vi "UpdateCVTFromSettingsCluster.vi"(8 "error in":errorcluster, 10 "SelectedProperty.Hierarchy":string[](array[string]), 11 "SettingsCluster":variant) -> (0 "error out":errorcluster)   [LabVIEW 2020]
uses:
  OnOffTypeDef.ctl
  UtilsLib/ClusterManipulation/GetClusterElementByName(Variant).vi
  UtilsLib/ClusterManipulation/GetClusterElementByName(DBL).vi
  CompressAndUpdate(Poly)/CompressAndUpdate(Enum).vi
  CompressAndUpdate(Poly)/CompressAndUpdate(Numeric).vi
  CompressAndUpdate(Poly)/CompressAndUpdate(String).vi
  CompressAndUpdate(Poly)/CompressAndUpdate(Path).vi
  UtilsLib/ClusterManipulation/GetClusterElementByName.lvlib
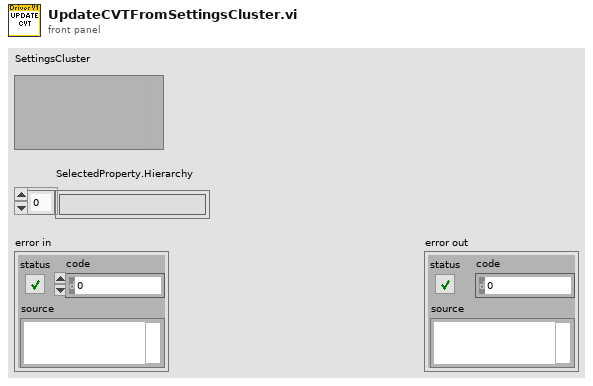
[diagram p1: front panel]
types:
  T1 = typedef "OnOffTypeDef.ctl" = enum16{"off", "on"}
  T2 = typedef "Type Descriptor Enumeration__ogtk.ctl" = enum8{"<Null>", "I8", "I16", "I32", "I64", "U8", "U16", "U32", "U64", "SGL", "DBL", "EXT", "CSG", "CDB", "CXT", "0x0F", "0x10", "0x11", "0x12", "0x13", "0x14", "Enum U8", "Enum U16", "Enum U32", "Enum U64", "SGL PQ", "DBL PQ", "EXT PQ", "CSG PQ", "CDB PQ", "CXT PQ", "0x1F", "0x20", "Boolean", "0x22", "0x23", "0x24", "0x25", "0x26", "0x27", "0x28", "0x29", "0x2A", "0x2B", "0x2C", "0x2D", "0x2E", "0x2F", "String", "0x31", "Path", "Pict", "0x34", "0x35", "0x36", "DAQ", "0x38", "0x39", "0x3A", "0x3B", "0x3C", "0x3D", "0x3E", "0x3F", "Array", "0x41", "0x42", "0x43", "0x44", "0x45", "0x46", "0x47", "0x48", "0x49", "0x4A", "0x4B", "0x4C", "0x4D", "0x4E", "0x4F", "Cluster", "0x51", "0x52", "Variant", "Waveform", "0x55", "0x56", "0x57", "0x58", "0x59", "0x5A", "0x5B", "0x5C", "0x5D", "0x5E", "0x5F", "0x60", "0x61", "0x62", "0x63", "0x64", "0x65", "0x66", "0x67", "0x68", "0x69", "0x6A", "0x6B", "0x6C", "0x6D", "0x6E", "0x6F", "Refnum"}
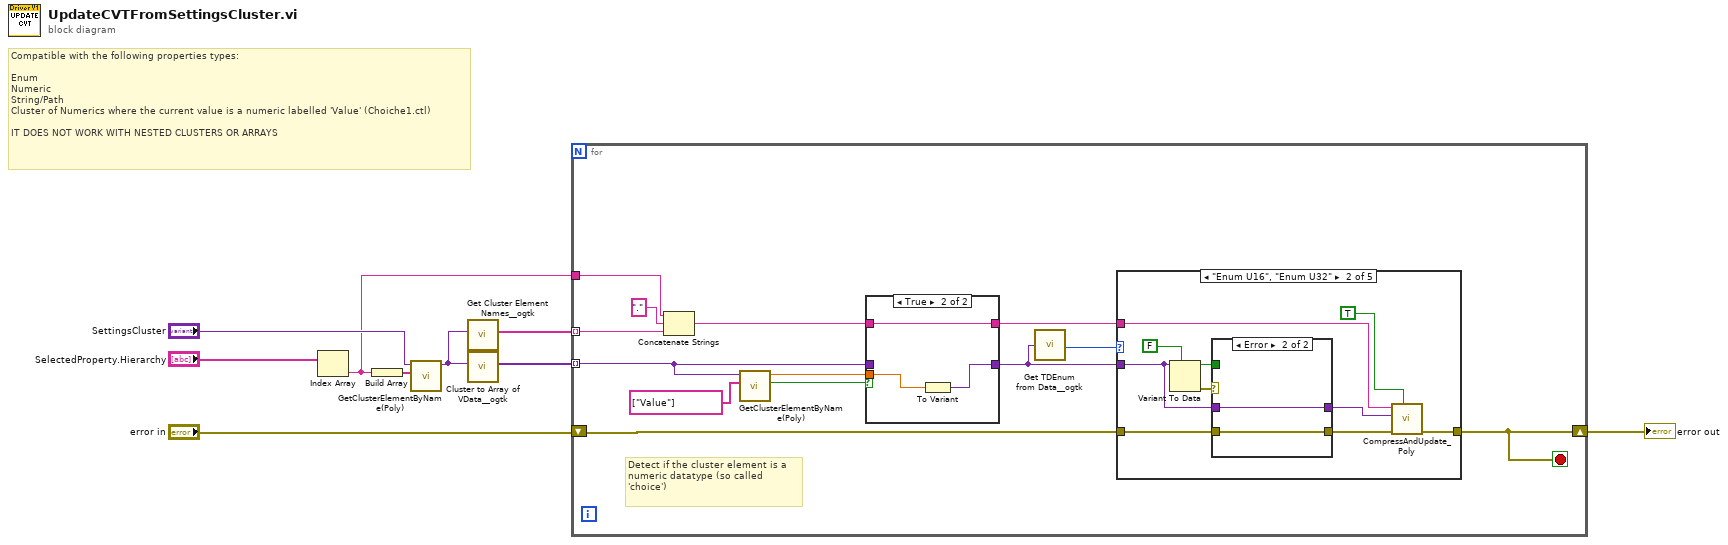
[diagram p0: block diagram]
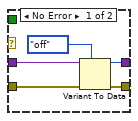
[diagram p3: hidden frame]
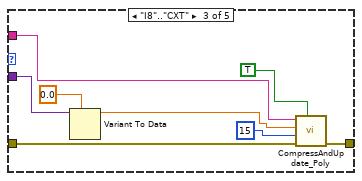
[diagram p4: hidden frame]
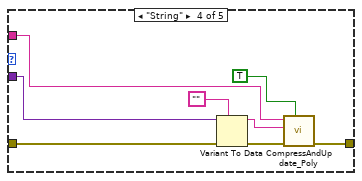
[diagram p5: hidden frame]
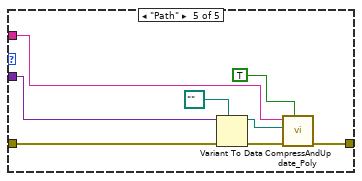
[diagram p6: hidden frame]
diagram:
  # "Compatible with the following properties types:\n\nEnum\nNumeric\nString/Path\nCluster of Numerics where the current value is a numeric labelled 'Value' (Choiche1.ctl)\n\nIT DOES NOT WORK WITH NESTED CLUSTERS OR ARRAYS"
  n1 = Index Array(array="SelectedProperty.Hierarchy") -> (element=w1:string)  [unwired: 1 in]
  n2 = Build Array(w1) -> (w2:string[])
  n3 = call-poly "GetClusterElementByName(Poly).vi"("ElementHierarchy"=w2, "Cluster"="SettingsCluster") -> ("Element"=w7:variant)  [unwired: 8 in, 1 out]
  n4 = call <userlib>:"Get Cluster Element Names__ogtk.vi"("Cluster"=w7) -> ("Element Names"=w4:string[])  [unwired: 9 in, 1 out]
  n5 = call <userlib>:"Cluster to Array of VData__ogtk.vi"("Cluster"=w7) -> ("Array of VData"=w3:variant[])  [unwired: 9 in, 1 out]
  n6 = for {
    tunnel: w4 -> [w20] mode=indexing
    tunnel: w1 -> [w21]
    tunnel: w3 -> [w11] mode=indexing
    shift-right: [w13] -> w6
    shift-left: "error in" -> [w15]
    stop <- w13 stop-if-true
    # "Detect if the cluster element is a numeric datatype (so called 'choice')"
    n7 = Concatenate Strings(w21, "." ("string"), w20) -> (w18:string)
    n8 = call-poly "GetClusterElementByName(Poly).vi"("ElementName"=string[] ["Value"], "Cluster"=w11) -> ("Found"=w19:bool, "ValueOut"=w16:dbl)  [unwired: 8 in]
    n9 = case shown="True" w19 {
      tunnel: w18 -> [w66 w67]
      tunnel: [w66 w67] -> w10
      tunnel: w16 -> [_ w69]
      tunnel: [w65 w68] -> w12
      tunnel: w11 -> [w65 _]
      frame False {
      }
      frame True {
        n10 = To Variant(anything=w69) -> (Variant=w68:variant)
      }
    }
    n11 = call <userlib>:"Get TDEnum from Data__ogtk.vi"("Data"=w12) -> ("Type Descriptor Enumeration"=w14:T2)  [unwired: 4 in]
    n12 = case shown="\"Enum U16\", \"Enum U32\"" w14 {
      tunnel: w12 -> [_ w31 w44 w54 w62]
      tunnel: w10 -> [_ w30 w47 w55 w63]
      tunnel: [w23 w27 w45 w51 w61] -> w13
      tunnel: w15 -> [w23 w25 w43 w50 w60]
      frame "<Null>", Default {
      }
      frame "Enum U16", "Enum U32" {
        n13 = Variant To Data(type=FALSE, Variant=w31) -> (data=w32:bool, error out=w33:errorcluster)  [unwired: 1 in]
        n14 = case shown="Error" w33 {
          tunnel: w32 -> [_ _]
          tunnel: [w36 w40] -> w29
          tunnel: w31 -> [w38 w40]
          tunnel: w25 -> [w35 w39]
          tunnel: [w34 w39] -> w24
          frame No Error {
            n15 = Variant To Data(error in=w35, type=OnOffTypeDef."off" ("Save"), Variant=w38) -> (data=w36:T1, error out=w34:errorcluster)
          }
          frame Error {
          }
        }
        n16 = call-poly "CompressAndUpdate_Poly.vi"("force CVT update (false)"=TRUE, "error in"=w24, "enum variant"=w29, "command or variable name"=w30) -> ("error out"=w27:errorcluster)  [unwired: 7 in]
      }
      frame "I8".."CXT" {
        n17 = Variant To Data(type=0.0, Variant=w44) -> (data=w41:dbl)  [unwired: 1 in, 1 out]
        n18 = call-poly "CompressAndUpdate_Poly.vi"("force CVT update (false)"=TRUE, "error in"=w43, "precision (6)"=i16 15, "Numeric"=w41, "command or variable name"=w47) -> ("error out"=w45:errorcluster)  [unwired: 6 in]
      }
      frame "String" {
        n19 = Variant To Data(error in=w50, type="", Variant=w54) -> (data=w52:string, error out=w49:errorcluster)
        n20 = call-poly "CompressAndUpdate_Poly.vi"("force CVT update (false)"=TRUE, "error in"=w49, "String"=w52, "command or variable name"=w55) -> ("error out"=w51:errorcluster)  [unwired: 7 in]
      }
      frame "Path" {
        n21 = Variant To Data(error in=w60, type=path "", Variant=w62) -> (data=w57:path, error out=w59:errorcluster)
        n22 = call-poly "CompressAndUpdate_Poly.vi"("force CVT update (false)"=TRUE, "error in"=w59, "Path"=w57, "command or variable name"=w63) -> ("error out"=w61:errorcluster)  [unwired: 7 in]
      }
    }
  }
  "error out" <- w6
